vi "SlopeAndOffset.vi"(8 "Offset":dbl, 9 "Slope":dbl, 10 "Index":i32, 11 "Data in":dbl[](array[numeric])) -> (3 "Data out":dbl[](array[numeric]))   [LabVIEW 2018, in "Controller (Host).lvlib"]
uses:
  Controller (Host).lvlib
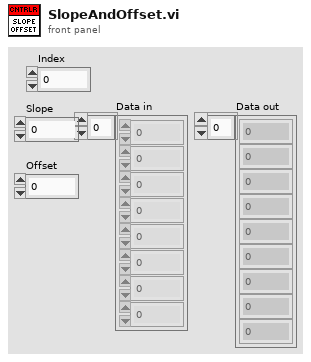
[diagram p1: front panel]
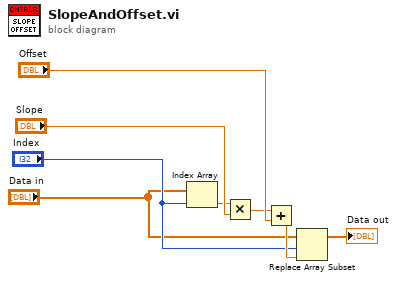
[diagram p0: block diagram]
diagram:
  n1 = Index Array(array="Data in", index="Index") -> (element=w1:dbl)
  n2 = Multiply(x=w1, y="Slope") -> (x*y=w3:dbl)
  n3 = Add(x=w3, y="Offset") -> (x+y=w7:dbl)
  n4 = Replace Array Subset(array="Data in", new element=w7, index="Index") -> (→"Data out":dbl[])
